vi "For Loop Iteration.vi"(4 "i":i32, 6 "N":i32) -> (5 "i (dup)":i32, 7 "Iteration":T1)   [LabVIEW 2021]
uses:
  For Loop Iteration Type.ctl
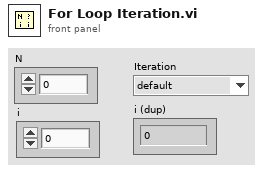
[diagram p1: front panel]
types:
  T1 = typedef "For Loop Iteration Type.ctl" = enum16{"default", "first", "last", "out of range"}
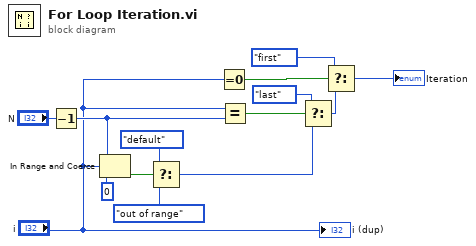
[diagram p0: block diagram]
diagram:
  n1 = Decrement(x="N") -> (x-1=w2:i32)
  n2 = In Range and Coerce(upper limit=w2, x="i", lower limit=0) -> (In Range?=w6:bool)  [unwired: 1 out]
  n3 = Select(t=For_Loop_Iteration_Type."default" ("f"), s=w6, f=For_Loop_Iteration_Type."out of range") -> (s? t:f=w3:T1)
  n4 = Equal To 0?(x="i") -> (x = 0?=w14:bool)
  n5 = Equal?(x="i", y=w2) -> (x = y?=w11:bool)
  n6 = Select(t=For_Loop_Iteration_Type."last" ("Iteration"), s=w11, f=w3) -> (s? t:f=w9:T1)
  n7 = Select(t=For_Loop_Iteration_Type."first" ("Iteration"), s=w14, f=w9) -> (s? t:f=→"Iteration":T1)
  "i (dup)" <- "i"
